vi "Get Case Structure Frame Index (by Name).vi"(8 "error in (no error)":errorcluster, 10 "element":string, 11 "CaseStructure in":refnum<vi>) -> (0 "error out":errorcluster, 1 "Found?":bool, 2 "Frame Index":i32, 3 "CaseStructure out":refnum<vi>)   [LabVIEW 2019, in "gRPC Scripting Tools.lvlib"]
uses:
  gRPC Scripting Tools.lvlib
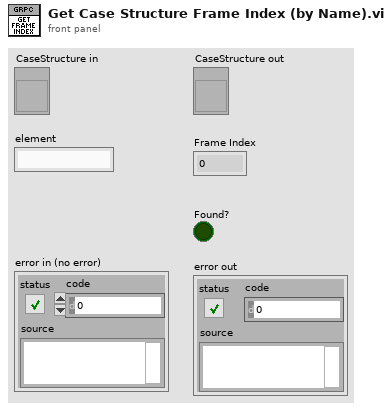
[diagram p1: front panel]
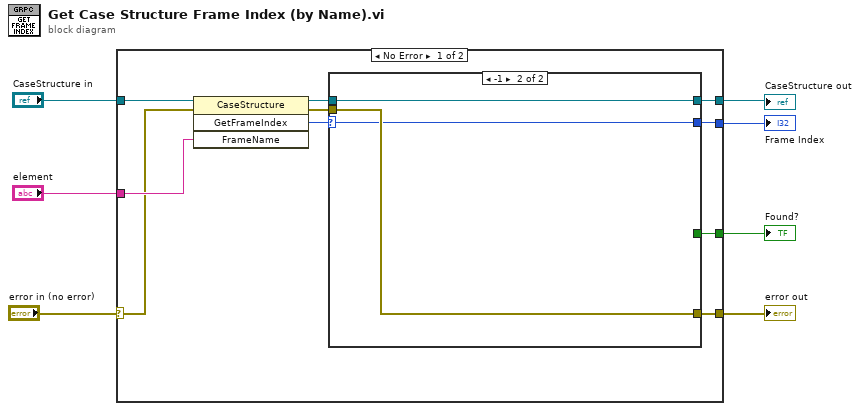
[diagram p0: block diagram]
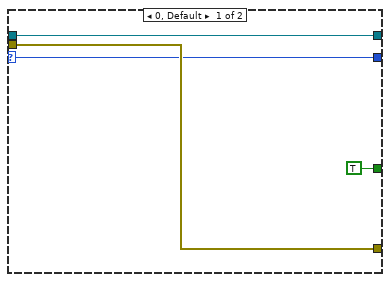
[diagram p2: hidden frame]
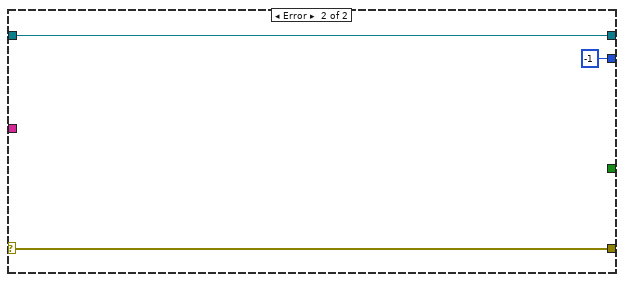
[diagram p3: hidden frame]
diagram:
  n1 = case shown="No Error" "error in (no error)" {
    selector: "error in (no error)" -> [w11 w27]
    tunnel: "CaseStructure in" -> [w17 w26]
    tunnel: [w16 w26] -> w6
    tunnel: [w15 w27] -> w5
    tunnel: "element" -> [w13 _]
    tunnel: [w9 _] -> w2
    tunnel: [w8 -1 ("GetFrameIndex")] -> w1
    frame No Error {
      n2 = invoke class="CaseStructure" method="GetFrameIndex"(reference=w17, error in=w11, "FrameName"=w13) -> (reference out=w14:refnum<vi>, error out=w12:errorcluster, "GetFrameIndex"=w10:i32)  [unwired: 1 in, 1 out]
      n3 = case shown="-1" w10 {
        selector: w10 -> [w18 w22]
        tunnel: [w20 w24] -> w16
        tunnel: [w19 w23] -> w15
        tunnel: w14 -> [w20 w24]
        tunnel: w12 -> [w19 w23]
        tunnel: [TRUE _] -> w9
        tunnel: [w18 w22] -> w8
        frame 0, Default {
        }
        frame -1 {
        }
      }
    }
    frame Error {
    }
  }
  "CaseStructure out" <- w6
  "error out" <- w5
  "Found?" <- w2
  "Frame Index" <- w1
